vi "ConvertDataFrom File (SubVI).vi"(0 "File Path Control":path) -> (10 "WrongFile?":bool, 11 "All bytes in file in HEX U8":u8[](array[numeric]) format="%02x", 14 "Header":u8[](array[numeric]) format="%.0x", 15 "sumHeader":u16 format="%.0x", 16 "Full Text File":u8[](array[numeric]) format="%.0x", 17 "Header":u16[](array[numeric]) format="%.0x")   [LabVIEW 2017]
panel:
  out "Size of Text File":i32
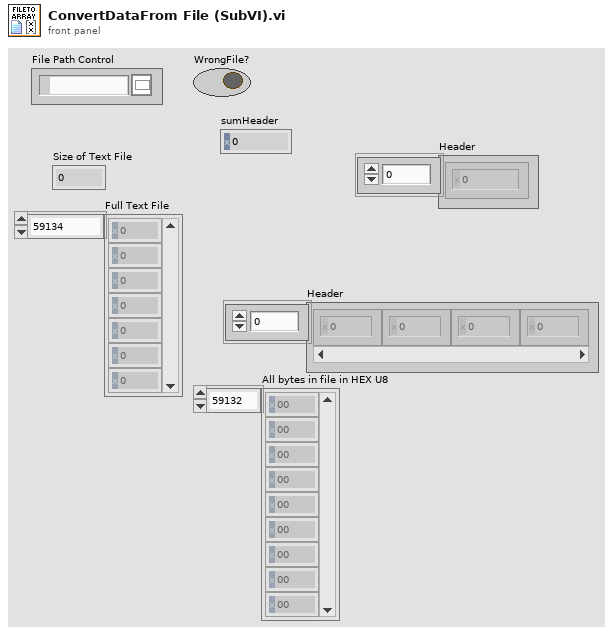
[diagram p1: front panel]
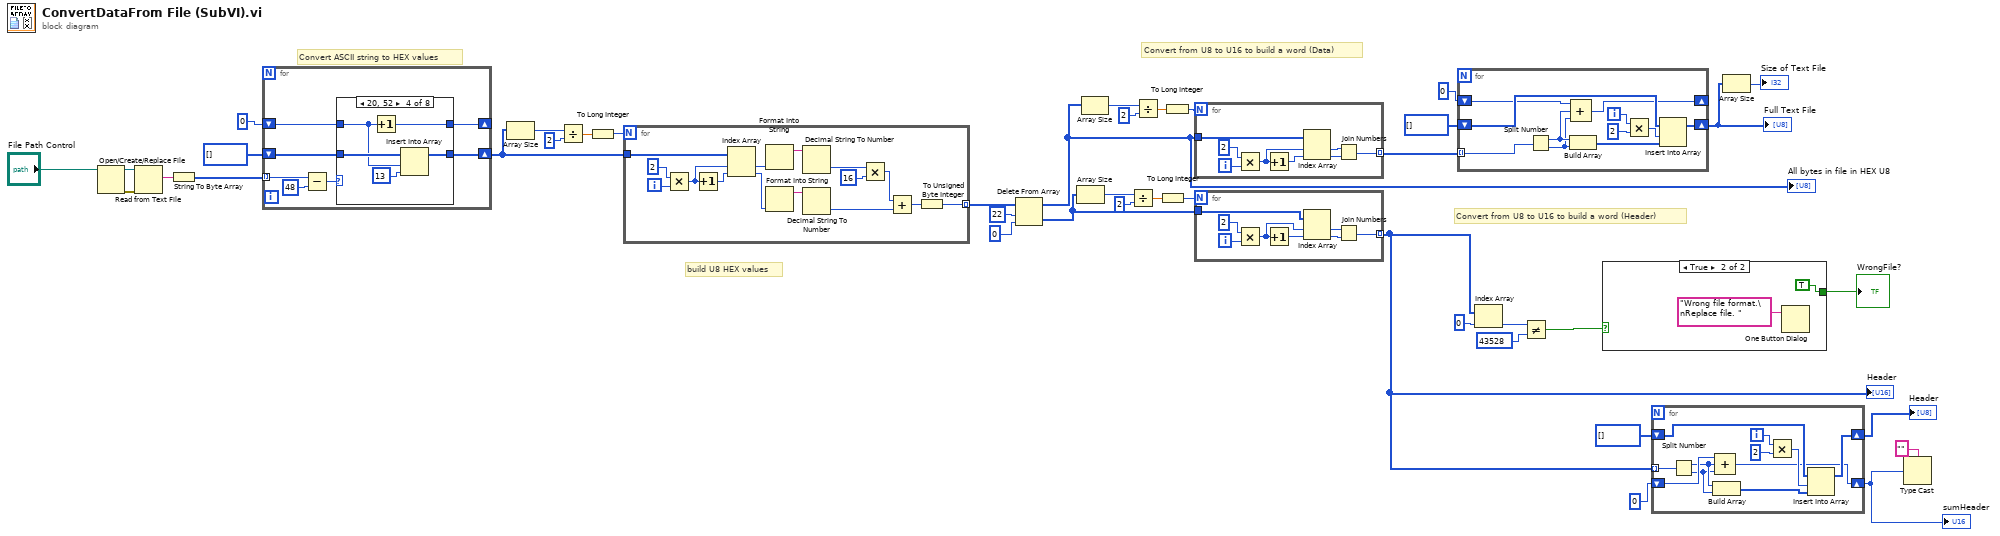
[diagram p0: block diagram]
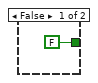
[diagram p2: hidden frame]
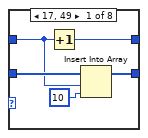
[diagram p3: hidden frame]
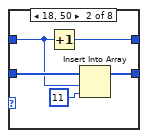
[diagram p4: hidden frame]
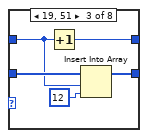
[diagram p5: hidden frame]
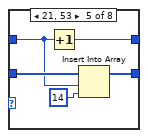
[diagram p6: hidden frame]
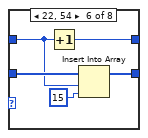
[diagram p7: hidden frame]
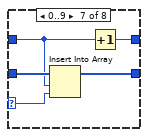
[diagram p8: hidden frame]
diagram:
  # "Convert from U8 to U16 to build a word (Header)"
  # "build U8 HEX values"
  # "Convert from U8 to U16 to build a word (Data)"
  # "Convert ASCII string to HEX values"
  n1 = Open/Create/Replace File(file path (use dialog)="File Path Control") -> (refnum out=w37:refnum<file>, error out=w38:errorcluster)  [unwired: 5 in, 1 out]
  n2 = Read from Text File(file (use dialog)=w37, error in=w38) -> (text=w7:string)  [unwired: 2 in, 3 out]
  n3 = String To Byte Array(string=w7) -> (unsigned byte array=w36:u8[])
  n4 = for {
    tunnel: w36 -> [w48] mode=indexing
    shift-right: [w44] -> w33
    shift-left: u8[] [] -> [w45]
    shift-right: [w43] -> _
    shift-left: 0 ("y") -> [w42]
    n5 = Subtract(x=w48, y=u8 48) -> (x-y=w46:u8)
    n6 = case shown="20, 52" w46 {
      selector: w46 -> [_ _ _ _ _ _ w82 _]
      tunnel: [w51 w56 w62 w66 w71 w76 w81 w85] -> w44
      tunnel: w45 -> [w53 w57 w63 w68 w73 w78 w83 w85]
      tunnel: [w49 w54 w59 w64 w69 w74 w79 w84] -> w43
      tunnel: w42 -> [w50 w55 w60 w65 w70 w75 w80 w84]
      frame 17, 49 {
        n7 = Increment(x=w50) -> (x+1=w49:i32)
        n8 = Insert Into Array(array=w53, index=w50, new element=u8 10) -> (w51:u8[])
      }
      frame 18, 50 {
        n9 = Increment(x=w55) -> (x+1=w54:i32)
        n10 = Insert Into Array(array=w57, index=w55, new element=u8 11) -> (w56:u8[])
      }
      frame 19, 51 {
        n11 = Increment(x=w60) -> (x+1=w59:i32)
        n12 = Insert Into Array(array=w63, index=w60, new element=u8 12) -> (w62:u8[])
      }
      frame 20, 52 {
        n13 = Increment(x=w65) -> (x+1=w64:i32)
        n14 = Insert Into Array(array=w68, index=w65, new element=u8 13) -> (w66:u8[])
      }
      frame 21, 53 {
        n15 = Increment(x=w70) -> (x+1=w69:i32)
        n16 = Insert Into Array(array=w73, index=w70, new element=u8 14) -> (w71:u8[])
      }
      frame 22, 54 {
        n17 = Increment(x=w75) -> (x+1=w74:i32)
        n18 = Insert Into Array(array=w78, index=w75, new element=u8 15) -> (w76:u8[])
      }
      frame 0..9 {
        n19 = Insert Into Array(array=w83, index=w80, new element=w82) -> (w81:u8[])
        n20 = Increment(x=w80) -> (x+1=w79:i32)
      }
      frame 240, Default {
      }
    }
  }
  n21 = Array Size(array=w33) -> (size(s)=w32:i32)
  n22 = Divide(x=w32, y=2) -> (x/y=w30:dbl)
  n23 = To Long Integer(number=w30) -> (32bit integer=w29:i32)
  n24 = for {
    N: w29 -> [_]
    tunnel: w33 -> [w100]
    tunnel: [w86] -> w28 mode=indexing
    i -> [w99]
    n25 = Multiply(x=2, y=w99) -> (x*y=w97:i32)
    n26 = Increment(x=w97) -> (x+1=w96:i32)
    n27 = Index Array(array=w100, index #1=w97, index #2=w96) -> (element #1=w89:u8, element #2=w88:u8)
    n28 = Format Into String(w89) -> (resulting string=w90:string)  [unwired: 3 in, 1 out]
    n29 = Format Into String(w88) -> (resulting string=w95:string)  [unwired: 3 in, 1 out]
    n30 = Decimal String To Number(string=w90) -> (number=w91:i32)  [unwired: 2 in, 1 out]
    n31 = Decimal String To Number(string=w95) -> (number=w94:i32)  [unwired: 2 in, 1 out]
    n32 = Multiply(x=w91, y=16) -> (x*y=w93:i32)
    n33 = Add(x=w93, y=w94) -> (x+y=w87:i32)
    n34 = To Unsigned Byte Integer(number=w87) -> (unsigned 8bit integer=w86:u8)
  }
  n35 = Delete From Array(array=w28, length=22, index=0) -> (deleted portion=w17:u8[], array with subset deleted=w39:u8[])
  "All bytes in file in HEX U8" <- w39
  n36 = Array Size(array=w17) -> (size(s)=w22:i32)
  n37 = Array Size(array=w39) -> (size(s)=w23:i32)
  n38 = Divide(x=w22, y=2) -> (x/y=w20:dbl)
  n39 = Divide(x=w23, y=2) -> (x/y=w25:dbl)
  n40 = To Long Integer(number=w20) -> (32bit integer=w19:i32)
  n41 = To Long Integer(number=w25) -> (32bit integer=w18:i32)
  n42 = for {
    N: w18 -> [_]
    tunnel: w39 -> [w105]
    tunnel: [w101] -> w8 mode=indexing
    i -> [w104]
    n43 = Multiply(x=2, y=w104) -> (x*y=w107:i32)
    n44 = Increment(x=w107) -> (x+1=w108:i32)
    n45 = Index Array(array=w105, index #1=w107, index #2=w108) -> (element #1=w103:u8, element #2=w102:u8)
    n46 = Join Numbers(hi=w103, lo=w102) -> ((hi.lo)=w101:u16)
  }
  n47 = for {
    N: w19 -> [_]
    tunnel: w17 -> [w113]
    tunnel: [w109] -> w6 mode=indexing
    i -> [w112]
    n48 = Multiply(x=2, y=w112) -> (x*y=w115:i32)
    n49 = Increment(x=w115) -> (x+1=w116:i32)
    n50 = Index Array(array=w113, index #1=w115, index #2=w116) -> (element #1=w111:u8, element #2=w110:u8)
    n51 = Join Numbers(hi=w111, lo=w110) -> ((hi.lo)=w109:u16)
  }
  "Header" <- w6
  n52 = for {
    tunnel: w8 -> [w127] mode=indexing
    shift-right: [w122] -> w11
    shift-left: u8[] [] -> [w121]
    shift-right: [w119] -> _
    shift-left: u16 0 -> [w120]
    i -> [w126]
    n53 = Split Number(x=w127) -> (hi(x)=w118:u8, lo(x)=w117:u8)
    n54 = Build Array(w118, w117) -> (w124:u8[])
    n55 = Compound Arithmetic op=ADD(w120, w118, w117) -> (w119:u16)
    n56 = Multiply(x=w126, y=2) -> (x*y=w123:i32)
    n57 = Insert Into Array(array=w121, index=w123, new element=w124) -> (w122:u8[])
  }
  "Full Text File" <- w11
  n58 = Index Array(array=w6, index=0) -> (element=w15:u16)
  n59 = Not Equal?(x=w15, y=u16 43528) -> (x != y?=w13:bool)
  n60 = case shown="True" w13 {
    tunnel: [FALSE TRUE] -> w41
    frame False {
    }
    frame True {
      n61 = One Button Dialog(message="Wrong file format.\nReplace file. ") -> ()  [unwired: 1 in, 1 out]
    }
  }
  "WrongFile?" <- w41
  n62 = for {
    tunnel: w6 -> [w141] mode=indexing
    shift-right: [w136] -> w2
    shift-left: u8[] [] -> [w135]
    shift-right: [w133] -> w1
    shift-left: u16 0 -> [w134]
    i -> [w140]
    n63 = Split Number(x=w141) -> (hi(x)=w132:u8, lo(x)=w131:u8)
    n64 = Build Array(w132, w131) -> (w138:u8[])
    n65 = Compound Arithmetic op=ADD(w134, w132, w131) -> (w133:u16)
    n66 = Multiply(x=w140, y=2) -> (x*y=w137:i32)
    n67 = Insert Into Array(array=w135, index=w137, new element=w138) -> (w136:u8[])
  }
  "sumHeader" <- w1
  "Header" <- w2
  n68 = Array Size(array=w11) -> (size(s)=→"Size of Text File":i32)
  n69 = Type Cast(type="", x=w1) -> ()  [unwired: 1 out]
